vi "dvp Vi Get Flip Horizontal State.vi"(10 "pFlipHorizontalState":i32, 11 "handle":u32) -> (2 "pFlipHorizontalState out":i32, 3 "function return":u32(ring))   [LabVIEW 2018, in "LabViewDVPCamera.lvlib"]
doc: "LabviewDvp2Api dvpStatus dvpViGetFlipHorizontalState(dvpHandle handle, BOOL *pFlipHorizontalState);"
uses:
  LabViewDVPCamera.lvlib
  LabViewDVPCamera/LabViewDVPCamera.dll
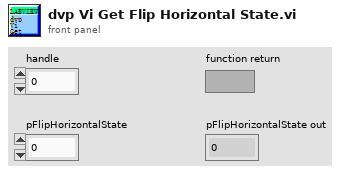
[diagram p1: front panel]
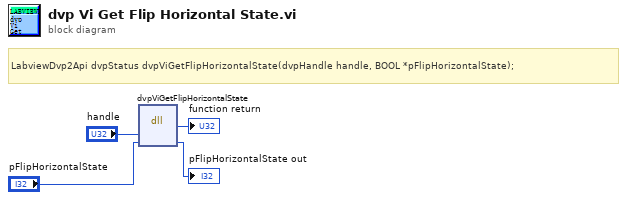
[diagram p0: block diagram]
diagram:
  # "LabviewDvp2Api dvpStatus dvpViGetFlipHorizontalState(dvpHandle handle, BOOL *pFlipHorizontalState);"
  n1 = dll-call lib="C:/Program Files (x86)/DVP2 Labview cn 64/Sample/LabViewDVPCamera/LabViewDVPCamera.*" fn="dvpViGetFlipHorizontalState"("handle"="handle", "pFlipHorizontalState"="pFlipHorizontalState") -> (→"function return":u32, "pFlipHorizontalState"=→"pFlipHorizontalState out":i32)  [unwired: 4 in, 2 out]
